vi "_io_read_ascii_or_bin_floatArray.vi"(7 "Timeout for chunked touts (-1: No chunked touts)":i32=-1, 8 "error in":errorcluster caption="error in (no error)", 11 "VISA resource name":refnum<visa-resource-name>) -> (0 "error out":errorcluster, 1 "Array Size":i32, 2 "Numbers out":dbl[](array[numeric]) format="%.2e", 3 "VISA resource name out":refnum<visa-resource-name>)   [LabVIEW 2020, in "Rohde&Schwarz RTx Oscilloscopes.lvlib" / "rsidr_core.lvlib"]
doc: "Queries array of floats that can be returned in ASCII format or in binary format. The array is always returned as the most-universal double array.\n- For <b>ASCII</b> format, the array numbers are decoded as comma-separated values.\n- For <b>Binary Format</b>, the numbers are decoded based on the session parameter <b>Bin Float Number Format</b>, usually float 32-bit (REAL,32), swapped endianess (instruments usually use low endian, LabVIEW uses big endian)."
uses:
  rsidr_core.lvlib
  type_Error_Codes.ctl
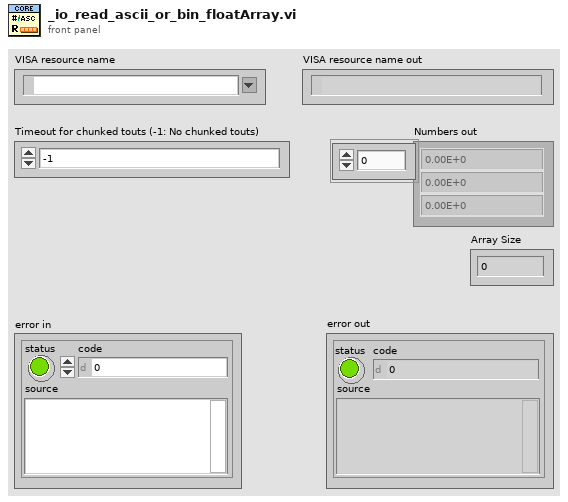
[diagram p1: front panel]
types:
  T1 = typedef "Rohde&Schwarz RTx Oscilloscopes.lvlib/rsidr_core.lvlib/type_Error_Codes.ctl" = enum16{"No_error", "VISA_err_ResourceNotFound", "VISA_err_Timeout", "VISA_warn_MoreDataAvailable", "RS_err_MissingCallback", "RS_err_InvalidAttribute", "RS_err_InvalidValue", "RS_err_UnknownResource", "RS_err_AlreadyInitialized", "RS_err_InstrumentStatus", "RS_err_BadRepCapName", "RS_err_TypesMismatch", "RS_err_ValueNotSupported", "RS_err_InvalidRngTable", "RS_err_IDqueryFail", "RS_err_UnexpResponse", "VISA_warn_ConfigNotLoaded", "RS_err_AttributeNotReadable", "RS_err_AttributeNotWritable", "RS_err_InstrumentType", "RS_err_InstrumentOption", "VISA_err_InvalidSize", "RS_err_ReliabilityIndicator", "VISA_warn_UnknownStatus", "VISA_warn_TermCharRead", "VISA_err_IO_error", "RS_err_FunctionNotSupported", "VISA_warn_QueueEmpty"}
  T2 = typedef "Rohde&Schwarz RTx Oscilloscopes.lvlib/rsidr_core.lvlib/type_Session_Data.ctl" = cluster{"IDN string":string, "Instrument FW":string, "Instr type":string, "Instr type for err. msg.":string, "Installed Options":string[], "Ignore Error Messages":string, "Logging params":variant, "OPC Timeout":i32, "VISA Timeout":i32, "STB Poll VISA Timeout":i32, "Additional Flags":i32, "Wait Before Read":i32, "Wait Before Write":i32, "Option String Flags":i32, "IO Segment Size":i64, "VISA Access Mode":T3, "Interface Type":T4, "OPC Wait Mode":T5, "Bin Float Number  Format":T6, "Bin Integer Number Format":T7, "Simulate":bool, "VXIcapable":bool, "Duplicate Session":bool, "Add LF to Write":bool, "Logging":bool, "Fast Sweep":bool, "Query Instrument Status":bool, "Check Range":bool, "Check Options":bool, "OPC-sync Attr Writes":bool, "OPC-sync Attr Queries":bool}
  T3 = typedef "Rohde&Schwarz RTx Oscilloscopes.lvlib/rsidr_core.lvlib/type_VisaAccessMode.ctl" = u16
  T4 = typedef "Rohde&Schwarz RTx Oscilloscopes.lvlib/rsidr_core.lvlib/type_InterfaceType.ctl" = enum16{"Unknown", "GPIB", "VXI", "GPIB_VXI", "ASRL", "PXI", "TCPIP", "USB", "SOCKET"}
  T5 = typedef "Rohde&Schwarz RTx Oscilloscopes.lvlib/rsidr_core.lvlib/type_OPC_Wait_Mode.ctl" = enum16{"STBpolling", "STBpollingSlow", "STBpollingSuperSlow", "ServiceRequest", "OPCquery"}
  T6 = typedef "Rohde&Schwarz RTx Oscilloscopes.lvlib/rsidr_core.lvlib/type_Binary_Float_Number_Format.ctl" = enum16{"Float_4_Bytes_Swapped", "Float_4_Bytes", "Double_8_Bytes_Swapped", "Double_8_Bytes"}
  T7 = typedef "Rohde&Schwarz RTx Oscilloscopes.lvlib/rsidr_core.lvlib/type_Binary_Integer_Number_Format.ctl" = enum16{"Int32_4_Bytes_Swapped", "Int32_4 Bytes", "Int16_2_Bytes_Swapped", "Int16_2_Bytes"}
  T8 = typedef "Rohde&Schwarz RTx Oscilloscopes.lvlib/rsidr_core.lvlib/_type_Return_Data_Type.ctl" = enum16{"BinData", "AsciiData", "EmptyAsciiData"}
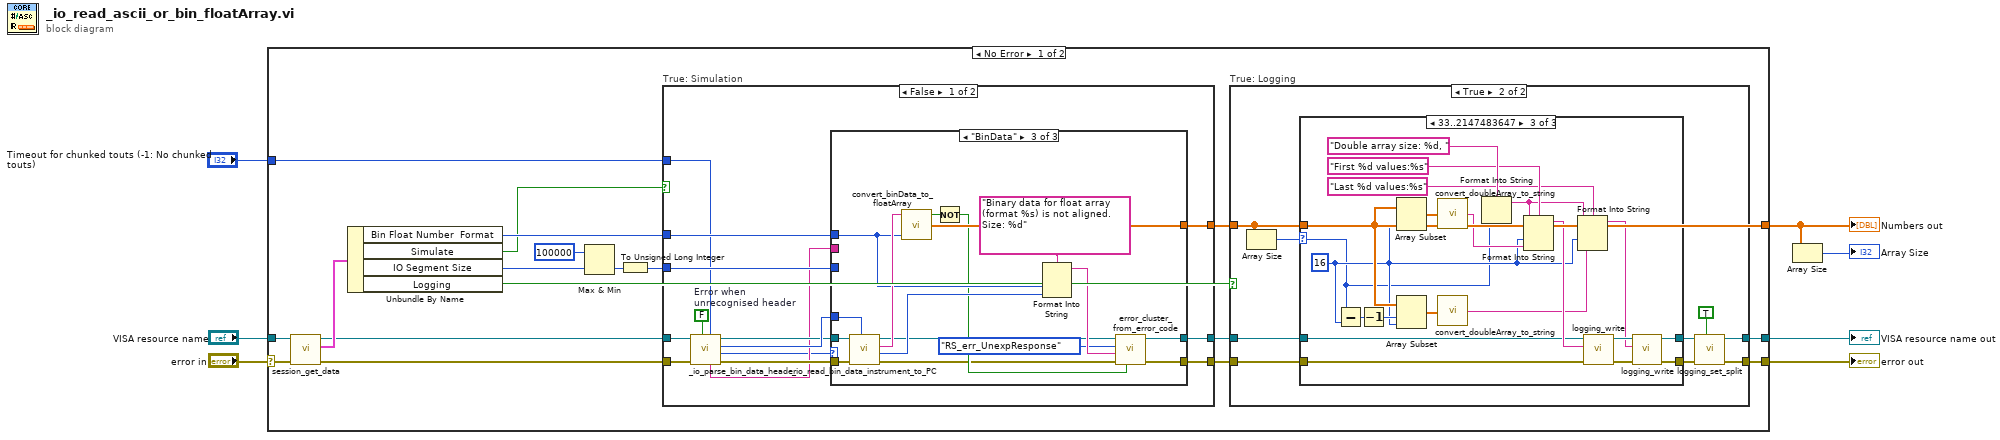
[diagram p0: block diagram]
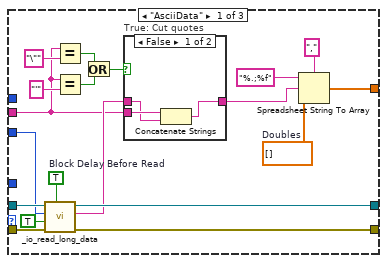
[diagram p2: hidden frame]
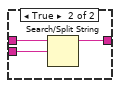
[diagram p3: hidden frame]
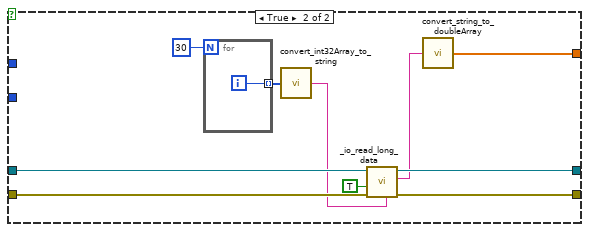
[diagram p5: hidden frame]
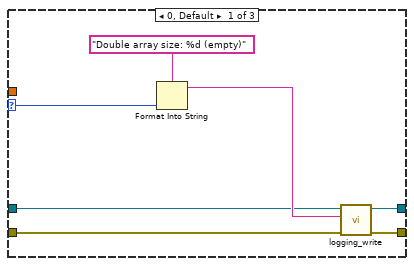
[diagram p7: hidden frame]
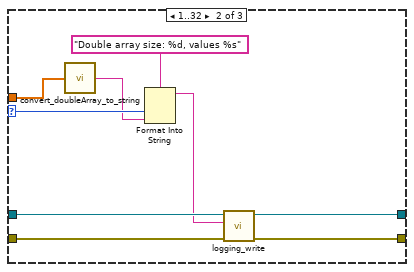
[diagram p8: hidden frame]
diagram:
  n1 = case shown="No Error" "error in" {
    selector: "error in" -> [w23 w143]
    tunnel: [w24 w142] -> w7
    tunnel: [w25 w143] -> w6
    tunnel: "VISA resource name" -> [w22 w142]
    tunnel: [w10 _] -> w2
    tunnel: "Timeout for chunked touts (-1: No chunked touts)" -> [w11 _]
    frame No Error {
      n2 = call "session_get_data.vi"("error in"=w23, "VISA resource name"=w22) -> ("error out"=w15:errorcluster, "Session User Data out"=w21:T2, "VISA resource name out"=w16:refnum<visa-resource-name>)  [unwired: 6 in, 1 out]
      n3 = Unbundle By Name(w21) -> ("Bin Float Number  Format"=w13:T6, "Simulate"=w12:bool, "IO Segment Size"=w17:i64, "Logging"=w20:bool)
      n4 = Max & Min(x=i64 100000 ("Max read bytes count (65536)"), y=w17) -> (min(x,y)=w18:i64)  [unwired: 1 out]
      n5 = To Unsigned Long Integer(number=w18) -> (unsigned 32bit integer=w14:u32)
      n6 = case "True: Simulation" shown="False" w12 {
        tunnel: w13 -> [w37 _]
        tunnel: w14 -> [w36 _]
        tunnel: w15 -> [w30 w92]
        tunnel: w16 -> [w29 w91]
        tunnel: [w33 w89] -> w9
        tunnel: [w32 w90] -> w8
        tunnel: [w31 w87] -> w10
        tunnel: w11 -> [w28 _]
        frame False {
          w39 = FALSE  # Error when unrecognised header
          n7 = call "_io_parse_bin_data_header.vi"("Timeout for chunked touts"=w28, "Error when unrecognised header (T)"=w39, "error in"=w30, "VISA resource name"=w29) -> ("error out"=w35:errorcluster, "Detected Data"=w26:T8, "Size of the bin data"=w38:i64, "VISA resource name out"=w34:refnum<visa-resource-name>, "Unparsed read portion"=w27:string)  [unwired: 3 in]
          n8 = case shown="\"BinData\"" w26 {
            tunnel: [w41 _ w79] -> w31
            tunnel: w34 -> [w57 w66 w82]
            tunnel: w35 -> [w58 w65 w80]
            tunnel: w38 -> [_ _ w81]
            tunnel: [w55 w66 w67] -> w33
            tunnel: [w56 w65 w68] -> w32
            tunnel: w37 -> [_ _ w72]
            tunnel: w36 -> [w54 _ _]
            tunnel: w27 -> [w43 _ _]
            frame "AsciiData" {
              w50 = TRUE  # Block Delay Before Read
              w53 = dbl[] []  # Doubles
              n9 = call "_io_read_long_data.vi"("Block Delay Before Read (F)"=w50, "error in"=w58, "Trim Response End (T)"=TRUE, "Max segment read bytes count (65536)"=w54, "VISA resource name"=w57) -> ("error out"=w56:errorcluster, "Read buffer"=w44:string, "VISA resource name out"=w55:refnum<visa-resource-name>)  [unwired: 3 in, 1 out]
              n10 = Equal?(x=w43, y="\"") -> (x = y?=w47:bool)
              n11 = Equal?(x=w43, y="'") -> (x = y?=w46:bool)
              n12 = Or(x=w47, y=w46) -> (x .or. y?=w45:bool)
              n13 = case "True: Cut quotes" shown="False" w45 {
                tunnel: w44 -> [w59 w64]
                tunnel: w43 -> [w60 w63]
                tunnel: [w61 w62] -> w42
                frame False {
                  n14 = Concatenate Strings(w60, w59) -> (w61:string)
                }
                frame True {
                  n15 = Search/Split String(string=w64, search string/char (-)=w63) -> (substring before match=w62:string)  [unwired: 1 in, 2 out]
                }
              }
              n16 = Spreadsheet String To Array(delimiter (Tab)=",", format string="%.;%f", spreadsheet string=w42, array type (2D Dbl)=w53) -> (array=w41:dbl[])
            }
            frame "EmptyAsciiData" {
            }
            frame "BinData" {
              n17 = call "_io_read_bin_data_instrument_to_PC.vi"("Direct Block Size in (Read and parse)"=w81, "error in"=w80, "VISA resource name"=w82) -> ("error out"=w70:errorcluster, "Data size Int64"=w73:i32, "Data out"=w78:string, "VISA resource name out"=w69:refnum<visa-resource-name>)  [unwired: 5 in]
              n18 = call "convert_binData_to_floatArray.vi"("Bin Float Number Format"=w72, "Bin Data"=w78) -> ("Numbers out"=w79:dbl[], "Bin Data Aligned"=w74:bool)  [unwired: 1 in, 1 out]
              n19 = Not(x=w74) -> (.not. x?=w71:bool)
              n20 = Format Into String(format string="Binary data for float array (format %s) is not aligned. Size: %d", w72, w73) -> (resulting string=w77:string)  [unwired: 2 in, 1 out]
              n21 = call "error_cluster_from_error_code.vi"("Error Creation Enabled (True)"=w71, "error in"=w70, "Error Message (\"\")"=w77, "Error Enum in"=type_Error_Codes."RS_err_UnexpResponse", "VISA resource name"=w69) -> ("error out"=w68:errorcluster, "VISA resource name out"=w67:refnum<visa-resource-name>)  [unwired: 5 in]
            }
          }
        }
        frame True {
          n22 = for {
            N: 30 -> [_]
            tunnel: [w93] -> w85 mode=indexing
            i -> [w93]
          }
          n23 = call "convert_int32Array_to_string.vi"("I32 array in"=w85) -> ("string out"=w84:string)  [unwired: 4 in]
          n24 = call "_io_read_long_data.vi"("Simulation read buffer (\"Simulation\")"=w84, "error in"=w92, "Trim Response End (T)"=TRUE, "VISA resource name"=w91) -> ("error out"=w90:errorcluster, "Read buffer"=w86:string, "VISA resource name out"=w89:refnum<visa-resource-name>)  [unwired: 4 in, 1 out]
          n25 = call "convert_string_to_doubleArray.vi"("string in"=w86) -> ("double array out"=w87:dbl[])  [unwired: 3 in, 1 out]
        }
      }
      n26 = case "True: Logging" shown="True" w20 {
        tunnel: w8 -> [w95 w99]
        tunnel: [w95 w103] -> w25
        tunnel: w9 -> [w94 w98]
        tunnel: [w94 w102] -> w24
        tunnel: w10 -> [_ w100]
        frame False {
        }
        frame True {
          n27 = Array Size(array=w100) -> (size(s)=w101:i32)
          n28 = case shown="33..2147483647" w101 {
            selector: w101 -> [w110 w119 w130]
            tunnel: w100 -> [_ w118 w141]
            tunnel: w99 -> [w108 w116 w128]
            tunnel: w98 -> [w107 w115 w127]
            tunnel: [w106 w114 w124] -> w97
            tunnel: [w105 w113 w123] -> w96
            frame 0, Default {
              n29 = Format Into String(format string="Double array size: %d (empty)", w110) -> (resulting string=w109:string)  [unwired: 2 in, 1 out]
              n30 = call "logging_write.vi"("error in"=w108, "String to write"=w109, "VISA resource name"=w107) -> ("error out"=w106:errorcluster, "VISA resource name out"=w105:refnum<visa-resource-name>)  [unwired: 7 in]
            }
            frame 1..32 {
              n31 = call "convert_doubleArray_to_string.vi"("double array in"=w118) -> ("string out"=w117:string)  [unwired: 4 in]
              n32 = Format Into String(format string="Double array size: %d, values %s", w119, w117) -> (resulting string=w112:string)  [unwired: 2 in, 1 out]
              n33 = call "logging_write.vi"("error in"=w116, "String to write"=w112, "VISA resource name"=w115) -> ("error out"=w114:errorcluster, "VISA resource name out"=w113:refnum<visa-resource-name>)  [unwired: 7 in]
            }
            frame 33..2147483647 {
              w132 = 16 ("length")
              n34 = Subtract(x=w130, y=w132) -> (x-y=w138:i32)
              n35 = Decrement(x=w138) -> (x-1=w137:i32)
              n36 = Array Subset(array=w141, length=w132) -> (w140:dbl[])  [unwired: 1 in]
              n37 = Array Subset(array=w141, index=w137, length=w132) -> (w139:dbl[])
              n38 = call "convert_doubleArray_to_string.vi"("double array in"=w140) -> ("string out"=w133:string)  [unwired: 4 in]
              n39 = call "convert_doubleArray_to_string.vi"("double array in"=w139) -> ("string out"=w121:string)  [unwired: 4 in]
              n40 = Format Into String(format string="Double array size: %d, ", w130) -> (resulting string=w129:string)  [unwired: 2 in, 1 out]
              n41 = Format Into String(format string="First %d values:%s", initial string=w129, w132, w133) -> (resulting string=w134:string)  [unwired: 1 in, 1 out]
              n42 = Format Into String(format string="Last %d values:%s", initial string=w129, w132, w121) -> (resulting string=w122:string)  [unwired: 1 in, 1 out]
              n43 = call "logging_write.vi"("error in"=w128, "String to write"=w134, "VISA resource name"=w127) -> ("error out"=w126:errorcluster, "VISA resource name out"=w125:refnum<visa-resource-name>)  [unwired: 7 in]
              n44 = call "logging_write.vi"("error in"=w126, "String to write"=w122, "VISA resource name"=w125) -> ("error out"=w124:errorcluster, "VISA resource name out"=w123:refnum<visa-resource-name>)  [unwired: 7 in]
            }
          }
          n45 = call "logging_set_split.vi"("Evaluate section error (F)"=TRUE, "error in"=w97, "VISA resource name"=w96) -> ("error out"=w103:errorcluster, "VISA resource name out"=w102:refnum<visa-resource-name>)  [unwired: 7 in]
        }
      }
    }
    frame Error {
    }
  }
  "error out" <- w6
  "VISA resource name out" <- w7
  "Numbers out" <- w2
  n46 = Array Size(array=w2) -> (size(s)=→"Array Size":i32)
